vi "calculate reverse power (percent of forward).vi"(1 "Reverse Power (dBm)":dbl, 2 "Forward Power (dBm)":dbl) -> (0 "Reverse Power (% of forward))":dbl)   [LabVIEW 2023]
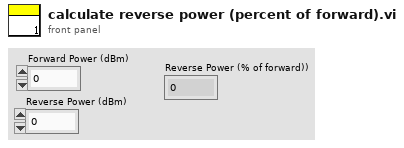
[diagram p1: front panel]
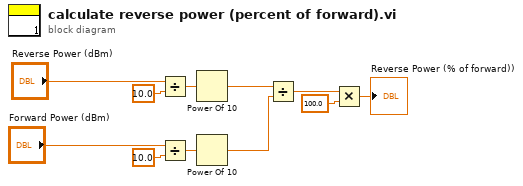
[diagram p0: block diagram]
diagram:
  n1 = Divide(x="Reverse Power (dBm)", y=10.0) -> (x/y=w6:dbl)
  n2 = Divide(x="Forward Power (dBm)", y=10.0) -> (x/y=w5:dbl)
  n3 = Power Of 10(x=w6) -> (10^x=w7:dbl)
  n4 = Power Of 10(x=w5) -> (10^x=w8:dbl)
  n5 = Divide(x=w7, y=w8) -> (x/y=w10:dbl)
  n6 = Multiply(x=w10, y=100.0) -> (x*y=→"Reverse Power (% of forward))":dbl)
